vi "Build_Header.vi"(9 "All_Bundled_Data_Brass Out":T1, 10 "ERD Number Array In":string[](array[string]), 11 "ERD Name Array In":string[](array[string])) -> (2 "ERD Name Array out 2":string[][](array[string]))   [LabVIEW 2021]
uses:
  type defs/All_Bundled_Data.ctl
  type defs/Version.ctl
  type defs/ERD_Always_Show.ctl
  type defs/Brass Matrix.ctl
  type defs/CSV_File_String_Arrays.ctl
  type defs/Redundant.ctl
  type defs/Algorithms.ctl
  type defs/ATC_Data.ctl
  type defs/Fault Table Array.ctl
  type defs/Fault_Table_Info.ctl
  Dryer Tool (Commercial 2)/JL Dryer Tool Support/type defs/ERD_RJ45.ctl
  Dryer Tool (Commercial 2)/JL Dryer Tool Support/type defs/ERD_Commercial_Laundry.ctl
  type defs/BootloaderVersion.ctl
panel:
  # "Wet Load Size"
  # "Dry Load Size"
  # "OOB"
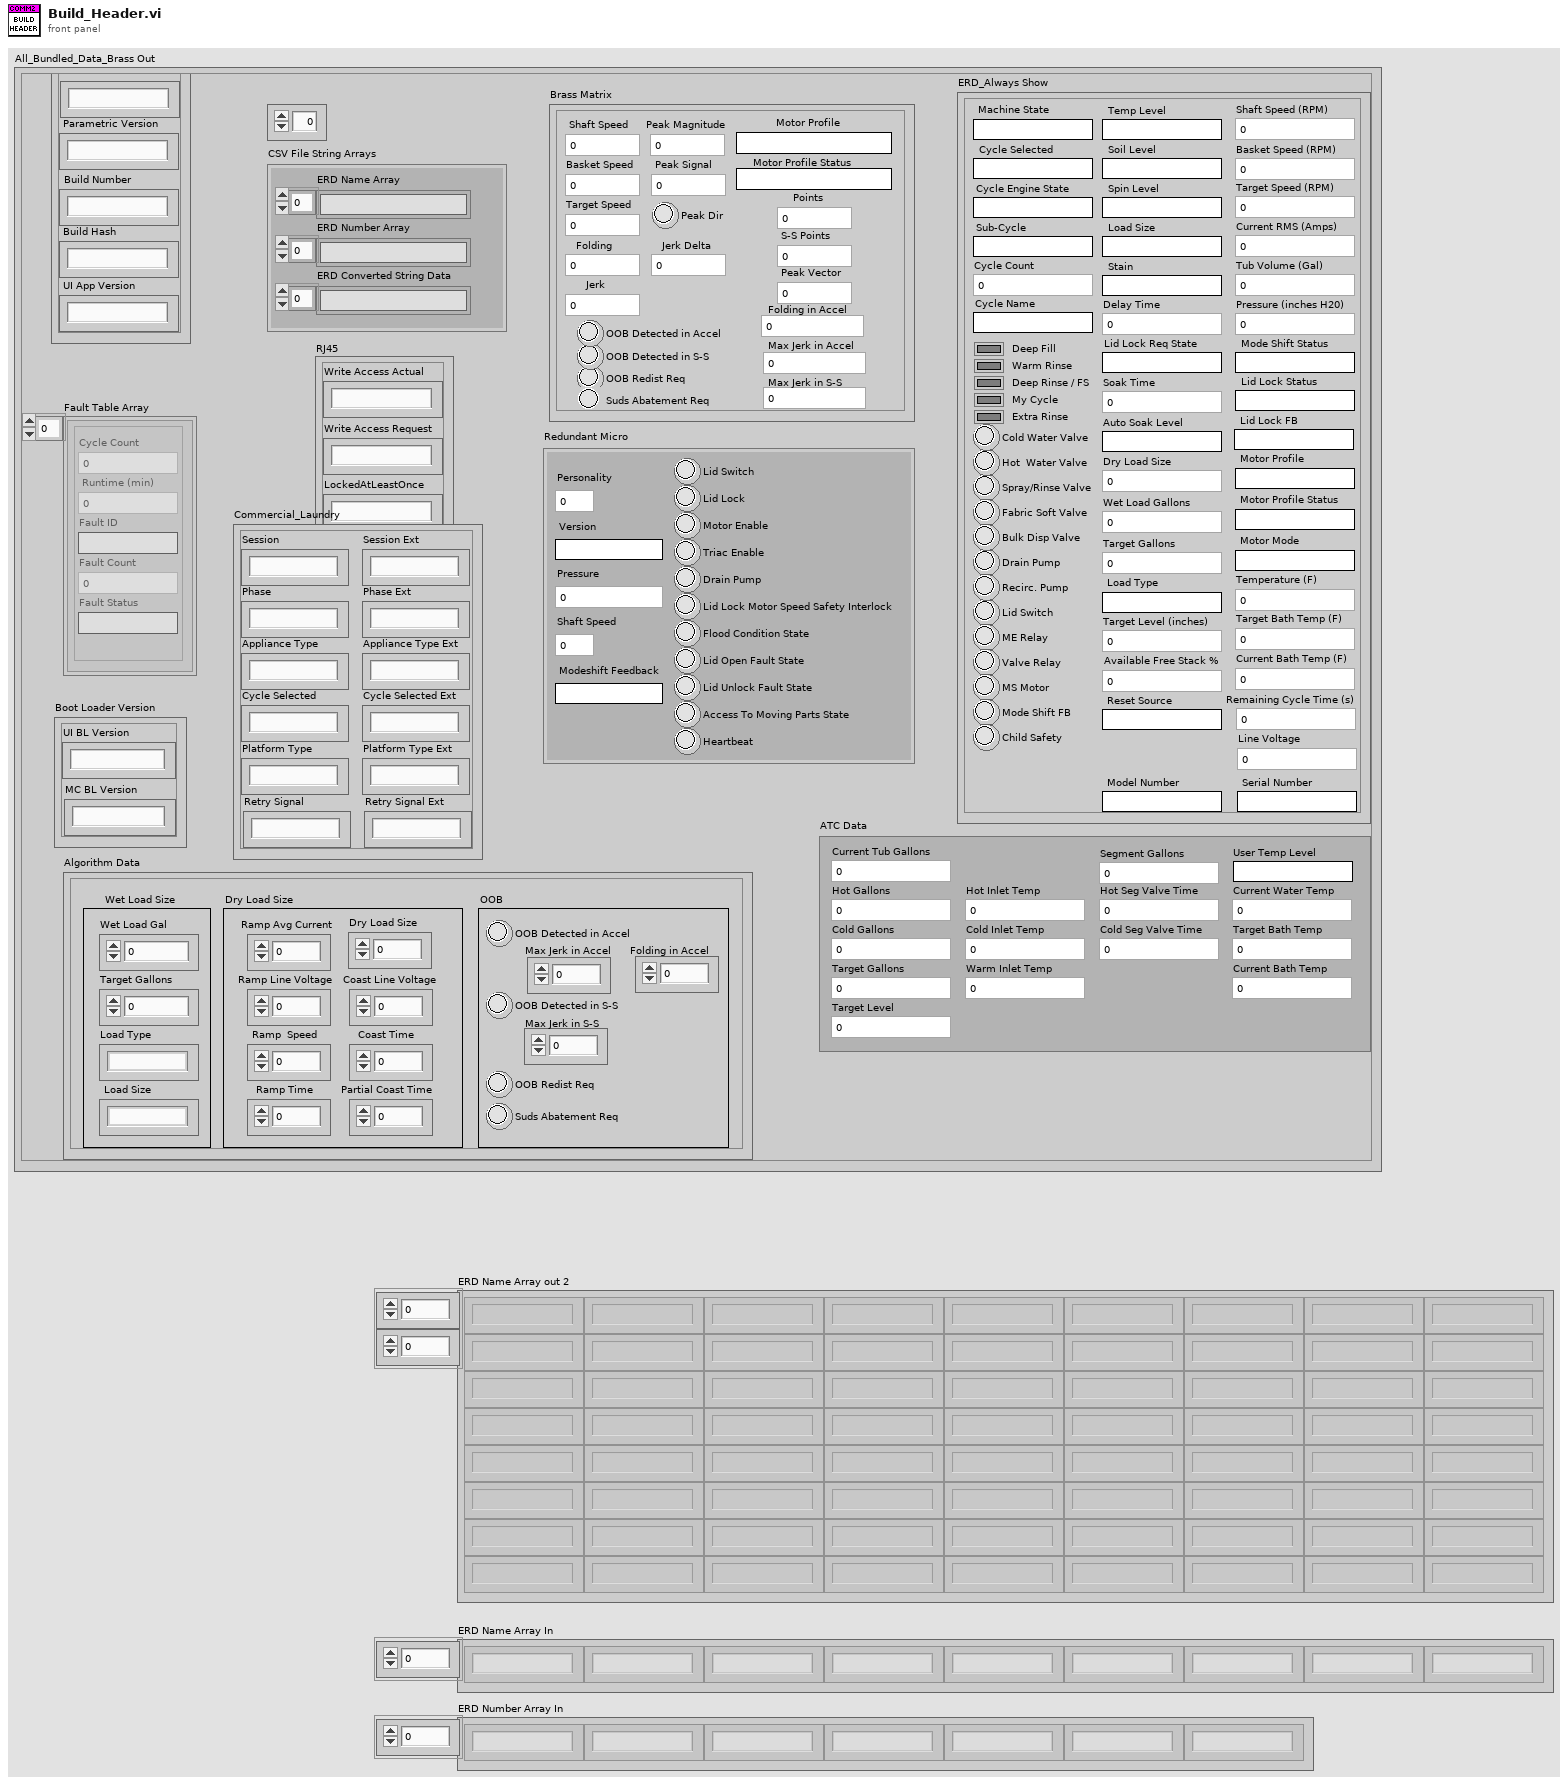
[diagram p1: front panel]
types:
  T1 = typedef "All_Bundled_Data.ctl" = cluster{"Software MC":T2, "ERD_Always Show":T3, "Personality Set":u8, "Brass Matrix":T4, "CSV File String Arrays":T5, "Redundant Micro":T6, "Algorithm Data":T7, "ATC Data":T8, "Fault Table Array ":T9, "RJ45":T11, "Commercial_Laundry":T12, "Boot Loader Version":T13}
  T2 = typedef "Version.ctl" = cluster{"Build Number":string, "Build Hash ":string, "Application Version":string, "Parametric Version":string, "UI App Version":string}
  T3 = typedef "ERD_Always_Show.ctl" = cluster{"Basket Speed (RPM)":u16, "Machine State":string, "Tub Volume (Gal)":dbl, "Pressure (inches H20)":dbl, "Lid Switch ":bool, "Current RMS (Amps)":dbl, "Cycle Selected":string, "Lid Lock Status":string, "Mode Shift Status":string, "Spray/Rinse Valve":bool, "Fabric Soft Valve":bool, "Drain Pump":bool, "Recirc. Pump":bool, "Cycle Engine State":string, "Hot  Water Valve":bool, "Cold Water Valve":bool, "Motor Profile":string, "Motor Profile Status":string, "Motor Mode":string, "ME Relay":bool, "Cycle Count":u32, "Deep Rinse / FS":bool, "My Cycle":bool, "Soil Level":string, "Spin Level":string, "Stain":string, "Temp Level":string, "Load Size":string, "Delay Time":u16, "Soak Time":u16, "Deep Fill":bool, "Warm Rinse":bool, "Auto Soak Level":string, "Extra Rinse":bool, "Wet Load Gallons":dbl, "Target Gallons":dbl, "Sub-Cycle":string, "Load Type":string, "Target Level (inches)":dbl, "Valve Relay":bool, "Dry Load Size":dbl, "Shaft Speed (RPM) ":u16, "MS Motor":bool, "Mode Shift FB":bool, "Target Bath Temp (F)":dbl, "Temperature (F)":dbl, "Current Bath Temp (F)":dbl, "Lid Lock FB":string, "Lid Lock Req State":string, "Remaining Cycle Time (s)":u32, "Available Free Stack %":u8, "Child Safety":bool, "Target Speed (RPM)":u16, "Reset Source":string, "Line Voltage":dbl, "Cycle Name":string, "Bulk Disp Valve":bool, "Model Number":string, "Serial Number":string}
  T4 = typedef "Brass Matrix.ctl" = cluster{"Shaft Speed":u16, "Folding":i32, "Jerk":i32, "Basket Speed":u16, "Target Speed":u16, "Peak Signal":u8, " Peak Magnitude":dbl, "Folding in Accel":i32, "Max Jerk in Accel":i32, "Max Jerk in S-S":i32, "Motor Profile Status":string, "Motor Profile":string, "OOB Redist Req":bool, "OOB Detected in S-S":bool, "OOB Detected in Accel":bool, "Suds Abatement Req ":bool, "Peak Dir":bool, "Peak Vector":dbl, "S-S Points":u8, "Points":u8, "Jerk Delta":i32}
  T5 = typedef "CSV_File_String_Arrays.ctl" = cluster{"ERD Number Array":string[], "ERD Name Array":string[], "ERD Converted String Data":string[]}
  T6 = typedef "Redundant.ctl" = cluster{"Version":string, "Personality":u8, "Pressure ":dbl, "Shaft Speed":u16, "Modeshift Feedback":string, "Lid Switch":bool, "Lid Lock":bool, "Triac Enable":bool, "Drain Pump":bool, "Lid Lock Motor Speed Safety Interlock":bool, "Flood Condition State":bool, "Lid Open Fault State":bool, "Access To Moving Parts State":bool, "Heartbeat":bool, "Motor Enable":bool, "Lid Unlock Fault State":bool}
  T7 = typedef "Algorithms.ctl" = cluster{"Wet Load Gal":dbl, "Target Gallons":dbl, "Load Type":string, "Load Size":string, "Coast Time":u16, "Ramp Time":u16, "Ramp  Speed":u16, "Ramp Avg Current":dbl, "OOB Redist Req":bool, "OOB Detected in S-S":bool, "Folding in Accel":i32, "Max Jerk in Accel":i32, "Max Jerk in S-S":i32, "OOB Detected in Accel":bool, "Partial Coast Time":u16, "Dry Load Size":dbl, "Ramp Line Voltage ":dbl, "Coast Line Voltage":dbl, "Suds Abatement Req ":bool}
  T8 = typedef "ATC_Data.ctl" = cluster{"Current Tub Gallons":dbl, "Hot Gallons":dbl, "Cold Gallons":dbl, "Target Gallons":dbl, "Current Water Temp":dbl, "Target Level":dbl, "Target Bath Temp":dbl, "Current Bath Temp ":dbl, "Cold Inlet Temp":dbl, "Hot Inlet Temp":dbl, "Warm Inlet Temp":dbl, "Hot Seg Valve Time":u16, "Cold Seg Valve Time ":u16, "User Temp Level":string, "Segment Gallons":dbl}
  T9 = typedef "Fault Table Array.ctl" = T10[]
  T10 = typedef "Fault_Table_Info.ctl" = cluster{"Cycle Count":u32, " Runtime (min) ":u32, "Fault Status":string, "Fault ID":string, "Fault Count":u16}
  T11 = typedef "ERD_RJ45.ctl" = cluster{"Write Access Actual":string, "Write Access Request":string, "LockedAtLeastOnce":string}
  T12 = typedef "ERD_Commercial_Laundry.ctl" = cluster{"Session":string, "Phase":string, "Appliance Type":string, "Cycle Selected":string, "Platform Type":string, "Retry Signal":string, "Session Ext":string, "Phase Ext":string, "Appliance Type Ext":string, "Cycle Selected Ext":string, "Platform Type Ext":string, "Retry Signal Ext":string}
  T13 = typedef "BootloaderVersion.ctl" = cluster{"UI BL Version":string, "MC BL Version":string}
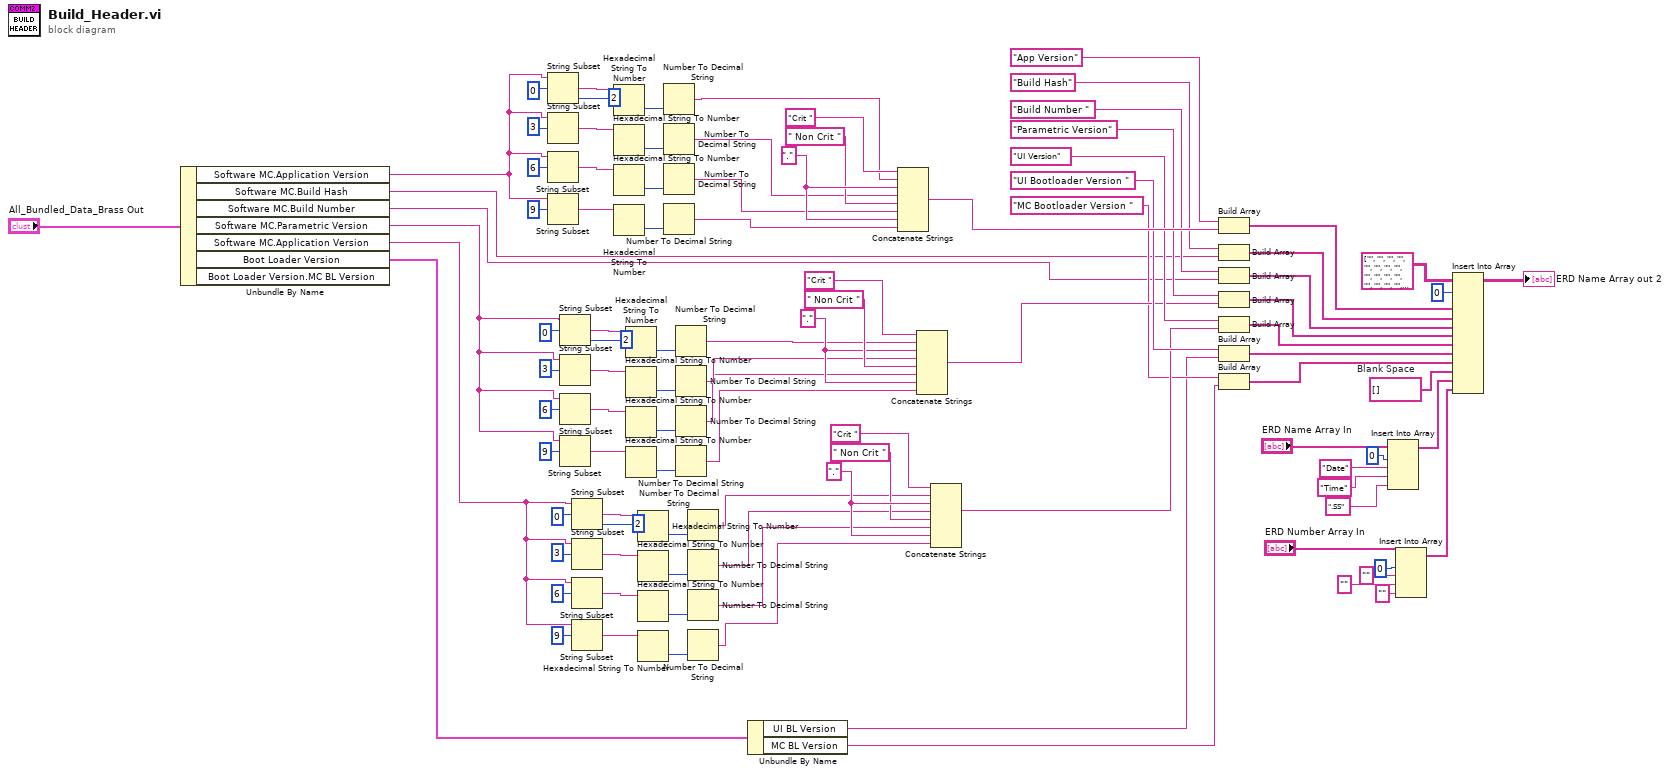
[diagram p0: block diagram]
diagram:
  w64 = string[] []  # Blank Space
  w96 = "." ("element")
  w97 = "." ("element")
  w102 = "." ("element")
  n1 = Unbundle By Name("All_Bundled_Data_Brass Out") -> ("Software MC.Application Version"=w44:string, "Software MC.Build Hash"=w39:string, "Software MC.Build Number"=w38:string, "Software MC.Parametric Version"=w24:string, "Software MC.Application Version"=w2:string, "Boot Loader Version"=w1:T13)  [unwired: 1 out]
  n2 = String Subset(string=w44, offset (0)=0 ("length (rest)"), length (rest)=2 ("length (rest)")) -> (substring=w45:string)
  n3 = String Subset(string=w44, offset (0)=3 ("length (rest)")) -> (substring=w49:string)  [unwired: 1 in]
  n4 = String Subset(string=w44, offset (0)=6 ("length (rest)")) -> (substring=w54:string)  [unwired: 1 in]
  n5 = String Subset(string=w44, offset (0)=9 ("length (rest)")) -> (substring=w55:string)  [unwired: 1 in]
  n6 = String Subset(string=w24, offset (0)=0 ("length (rest)"), length (rest)=2 ("length (rest)")) -> (substring=w37:string)
  n7 = String Subset(string=w24, offset (0)=3 ("length (rest)")) -> (substring=w33:string)  [unwired: 1 in]
  n8 = String Subset(string=w24, offset (0)=6 ("length (rest)")) -> (substring=w28:string)  [unwired: 1 in]
  n9 = String Subset(string=w24, offset (0)=9 ("length (rest)")) -> (substring=w27:string)  [unwired: 1 in]
  n10 = String Subset(string=w2, offset (0)=0 ("length (rest)"), length (rest)=2 ("length (rest)")) -> (substring=w7:string)
  n11 = String Subset(string=w2, offset (0)=3 ("length (rest)")) -> (substring=w11:string)  [unwired: 1 in]
  n12 = String Subset(string=w2, offset (0)=6 ("length (rest)")) -> (substring=w16:string)  [unwired: 1 in]
  n13 = String Subset(string=w2, offset (0)=9 ("length (rest)")) -> (substring=w17:string)  [unwired: 1 in]
  n14 = Hexadecimal String To Number(string=w45) -> (number=w50:u32)  [unwired: 2 in, 1 out]
  n15 = Hexadecimal String To Number(string=w49) -> (number=w51:u32)  [unwired: 2 in, 1 out]
  n16 = Hexadecimal String To Number(string=w54) -> (number=w52:u32)  [unwired: 2 in, 1 out]
  n17 = Hexadecimal String To Number(string=w55) -> (number=w53:u32)  [unwired: 2 in, 1 out]
  n18 = Hexadecimal String To Number(string=w37) -> (number=w32:u32)  [unwired: 2 in, 1 out]
  n19 = Hexadecimal String To Number(string=w33) -> (number=w31:u32)  [unwired: 2 in, 1 out]
  n20 = Hexadecimal String To Number(string=w28) -> (number=w30:u32)  [unwired: 2 in, 1 out]
  n21 = Hexadecimal String To Number(string=w27) -> (number=w29:u32)  [unwired: 2 in, 1 out]
  n22 = Hexadecimal String To Number(string=w7) -> (number=w12:u32)  [unwired: 2 in, 1 out]
  n23 = Hexadecimal String To Number(string=w11) -> (number=w13:u32)  [unwired: 2 in, 1 out]
  n24 = Hexadecimal String To Number(string=w16) -> (number=w14:u32)  [unwired: 2 in, 1 out]
  n25 = Hexadecimal String To Number(string=w17) -> (number=w15:u32)  [unwired: 2 in, 1 out]
  n26 = Number To Decimal String(number=w50) -> (decimal integer string=w43:string)  [unwired: 1 in]
  n27 = Number To Decimal String(number=w51) -> (decimal integer string=w42:string)  [unwired: 1 in]
  n28 = Number To Decimal String(number=w52) -> (decimal integer string=w41:string)  [unwired: 1 in]
  n29 = Number To Decimal String(number=w53) -> (decimal integer string=w40:string)  [unwired: 1 in]
  n30 = Number To Decimal String(number=w32) -> (decimal integer string=w23:string)  [unwired: 1 in]
  n31 = Number To Decimal String(number=w31) -> (decimal integer string=w22:string)  [unwired: 1 in]
  n32 = Number To Decimal String(number=w30) -> (decimal integer string=w21:string)  [unwired: 1 in]
  n33 = Number To Decimal String(number=w29) -> (decimal integer string=w20:string)  [unwired: 1 in]
  n34 = Number To Decimal String(number=w12) -> (decimal integer string=w6:string)  [unwired: 1 in]
  n35 = Number To Decimal String(number=w13) -> (decimal integer string=w5:string)  [unwired: 1 in]
  n36 = Number To Decimal String(number=w14) -> (decimal integer string=w4:string)  [unwired: 1 in]
  n37 = Number To Decimal String(number=w15) -> (decimal integer string=w3:string)  [unwired: 1 in]
  n38 = Unbundle By Name(w1) -> ("UI BL Version"=w59:string, "MC BL Version"=w58:string)
  n39 = Concatenate Strings("Crit " ("element"), w43, w102, w42, " Non Crit " ("element"), w41, w102, w40) -> (w90:string)
  n40 = Concatenate Strings("Crit " ("element"), w23, w97, w22, " Non Crit " ("element"), w21, w97, w20) -> (w73:string)
  n41 = Concatenate Strings("Crit " ("element"), w6, w96, w5, " Non Crit " ("element"), w4, w96, w3) -> (w74:string)
  n42 = Build Array("App Version" ("new element/subarray"), w90) -> (w92:string[])
  n43 = Build Array("Build Hash" ("new element/subarray"), w39) -> (w88:string[])
  n44 = Build Array("Build Number " ("new element/subarray"), w38) -> (w86:string[])
  n45 = Build Array("Parametric Version" ("new element/subarray"), w73) -> (w85:string[])
  n46 = Build Array("UI Version" ("new element/subarray"), w74) -> (w84:string[])
  n47 = Build Array("UI Bootloader Version " ("new element/subarray"), w59) -> (w72:string[])
  n48 = Build Array("MC Bootloader Version " ("new element/subarray"), w58) -> (w61:string[])
  n49 = Insert Into Array(array="ERD Name Array In", index=0, new element #1="Date", new element #2="Time", new element #3=".SS" ("new element/subarray")) -> (w63:string[])
  n50 = Insert Into Array(array="ERD Number Array In", index=0, new element #1="" ("new element/subarray"), new element #2="" ("new element/subarray"), new element #3="" ("new element/subarray")) -> (w62:string[])
  n51 = Insert Into Array(array=string[][] [["", "", "", "", "", "", "", "", "", "", "", "", "", "", "", "", "", "", "", "", "", "", "", "", "", "", "", "", "", "", "", "", "", "", "", "", "", "", "", "", "0"]] ("Array Ini"), index (row)=0, new element #1=w92, new element #2=w88, new element #3=w86, new element #4=w85, new element #5=w84, new element #6=w72, new element #7=w61, new element #8=w64, new element #9=w63, new element #10=w62) -> (→"ERD Name Array out 2":string[][])  [unwired: 1 in]
